vi "Signature Instance from Algorithm.vi"(10 "error in (no error)":errorcluster, 11 "Signature Algorithm":T1) -> (2 "error out":errorcluster, 3 "Signature":refnum<class "Signature.lvclass">)   [LabVIEW 2015, in "JWT.lvlib"]
uses:
  JWT.lvlib
  lv-crypto/Crypto/Signatures/None/None.lvclass
  lv-crypto/Crypto/Signatures/HMAC/HMAC.lvclass
  lv-crypto/Crypto/Hashes/SHA-256/SHA-256.lvclass
  Signature Algorithms.ctl
  lv-crypto/Crypto/Signature/Signature.lvclass
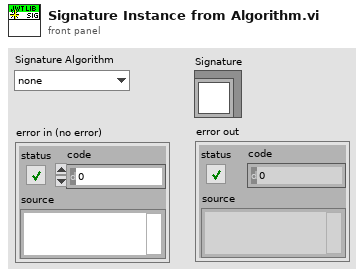
[diagram p1: front panel]
types:
  T1 = typedef "JWT.lvlib/Signature Algorithms.ctl" = enum16{"none", "HS256"}
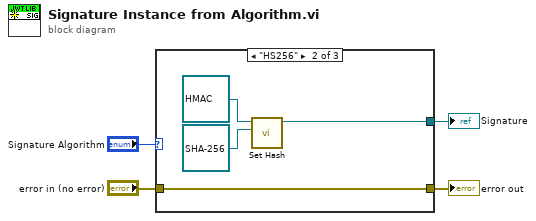
[diagram p0: block diagram]
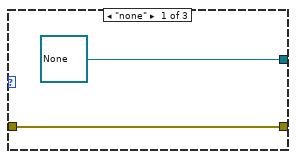
[diagram p2: hidden frame]
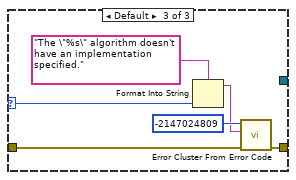
[diagram p3: hidden frame]
diagram:
  n1 = case shown="\"HS256\"" "Signature Algorithm" {
    selector: "Signature Algorithm" -> [_ _ w13]
    tunnel: [refnum<class "None.lvclass"> refnum ("Crypto.lvlibp:None.lvclass") w7 _] -> w3
    tunnel: "error in (no error)" -> [w5 w9 w15]
    tunnel: [w5 w9 w14] -> w1
    frame "none" {
    }
    frame "HS256" {
      n2 = call "Set Hash.vi"("Hash"=refnum<class "SHA-256.lvclass"> refnum ("Crypto.lvlibp:SHA-256.lvclass"), "HMAC in"=refnum<class "HMAC.lvclass"> refnum ("Crypto.lvlibp:HMAC.lvclass")) -> ("HMAC out"=w7:refnum<class "HMAC.lvclass">)  [unwired: 8 in, 1 out]
    }
    frame Default {
      n3 = Format Into String(format string="The \"%s\" algorithm doesn't have an implementation specified.", w13) -> (resulting string=w12:string)  [unwired: 2 in, 1 out]
      n4 = call <vilib>:"Error Cluster From Error Code.vi"("error in (no error)"=w15, "error message (\"\")"=w12, "error code (0)"=-2147024809) -> ("error out"=w14:errorcluster)  [unwired: 6 in]
    }
  }
  "error out" <- w1
  "Signature" <- w3
